vi "example 3 - subpanel1.vi"() -> ()   [LabVIEW 2020]
panel:
  in  "myNumber":dbl
  out "greater":bool caption="Greater than 5 ?"
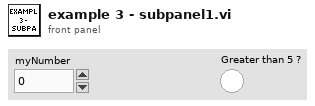
[diagram p1: front panel]
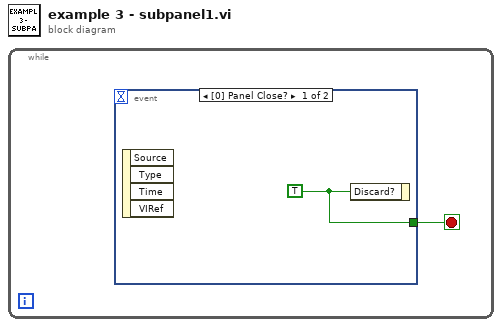
[diagram p0: block diagram]
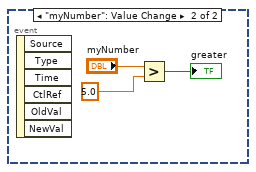
[diagram p2: hidden frame]
diagram:
  n1 = while {
    stop <- w1 stop-if-true
    n2 = event shown="[0] Panel Close?" {
      selector: _ -> [_ _]
      dyn-events: _ -> [_ _]
      timeout: _ -> [_ _]
      tunnel: [w2 _] -> w1
      event Panel Close? {
        w2 = TRUE
        n3 = event-data() -> ()  [unwired: 1 in, 4 out]
        n4 = event-data("Discard?"=w2) -> ()  [unwired: 1 in, 1 out]
      }
      event "myNumber": Value Change {
        n5 = event-data() -> ()  [unwired: 1 in, 6 out]
        n6 = Greater?(x="myNumber", y=5.0) -> (0:→"greater":bool)
      }
    }
  }
